vi "Try Step.vi"(8 "error in (no error)":errorcluster, 11 "Future in":refnum<class "Future.lvclass">) -> (0 "error out":errorcluster, 2 "Ready":bool, 3 "Future out":refnum<class "Future.lvclass">)   [LabVIEW 2020, in "Promises.lvlib" / "Future.lvclass"]
doc: "This performs a step of Promise chaining if a value is available and returns as quickly as possible. This VI does no waiting to see if a Promise has been resolved and is meant to return as quickly as possible. Once the last Promise has been resolved, Ready will return as True signifying that a call to <b>Wait.vi</b> will not have to wait for resolution.\n\nNormally promise chaining only happens within a <b>Wait.vi</b> call but this VI allows \"polling\" the value transfer between Promises and return the status of the last Promise in the chain. (Or the status of the only Promise if no <b>Then.vi</b> chaining has been setup."
uses:
  Future.lvclass
  Future.lvclass/Future.ctl
  Promise/Promise.lvclass/Promise.ctl
  Create.vi
  Promise/Promise.lvclass
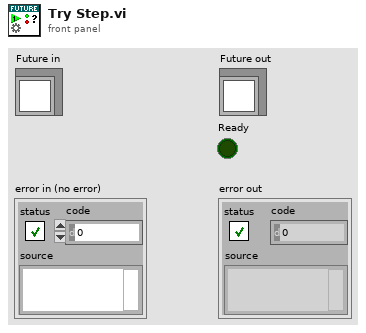
[diagram p1: front panel]
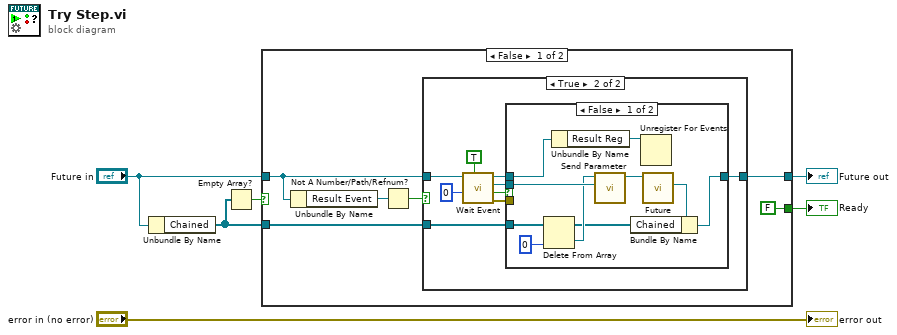
[diagram p0: block diagram]
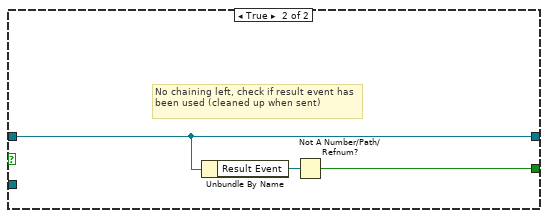
[diagram p4: hidden frame]
diagram:
  n1 = Unbundle By Name("Future in") -> ("Chained"=w2:refnum<class "Promise.lvclass">[])
  n2 = Empty Array?(array=w2) -> (empty?=w3:bool)
  n3 = case shown="False" w3 {
    tunnel: "Future in" -> [w9 w34]
    tunnel: [w12 w34] -> w4
    tunnel: w2 -> [w11 _]
    tunnel: [FALSE w35] -> w1
    frame False {
      n4 = Unbundle By Name(w9) -> ("Result Event"=w8:refnum<user-event>)
      n5 = Not A Number/Path/Refnum?(number/path/refnum=w8) -> (NaN/Path/Refnum?=w7:bool)
      n6 = case shown="True" w7 {
        tunnel: [w13 w17] -> w12
        tunnel: w11 -> [_ w16]
        tunnel: w9 -> [w13 w14]
        frame False {
          # "Han't been fired yet"
        }
        frame True {
          n7 = call "Wait Event.vi"("Keep Event Reg (F)"=TRUE, "Timeout mS (-1)"=0, "Future in"=w14) -> ("error out"=w20:errorcluster, "Timed Out"=w15:bool, "Value"=w18:refnum<class>, "Future out"=w19:refnum<class "Future.lvclass">)  [unwired: 5 in]
          n8 = case shown="False" w15 {
            tunnel: w19 -> [w32 w33]
            tunnel: w18 -> [w30 _]
            tunnel: [w24 w33] -> w17
            tunnel: w16 -> [w28 _]
            tunnel: w20 -> [_ _]
            frame False {
              n9 = Delete From Array(array=w28, index=0) -> (deleted portion=w26:refnum<class "Promise.lvclass">, array with subset deleted=w23:refnum<class "Promise.lvclass">[])  [unwired: 1 in]
              n10 = Unbundle By Name(w32) -> ("Result Reg"=w31:refnum<event-registration>)
              n11 = call "Send Parameter.vi"("Parameter"=w30, "Promise in"=w26) -> ("Promise out"=w29:refnum<class "Promise.lvclass">)  [unwired: 8 in, 1 out]
              n12 = Unregister For Events(event registration refnum=w31) -> ()  [unwired: 1 in, 1 out]
              n13 = call "Future.vi"("Promise in"=w29) -> ("Future"=w25:refnum<class "Future.lvclass">)  [unwired: 9 in, 1 out]
              n14 = Bundle By Name(cluster=w25, "Chained"=w23) -> (w24:refnum<class "Future.lvclass">)
            }
            frame True {
            }
          }
        }
      }
    }
    frame True {
      # "No chaining left, check if result event has been used (cleaned up when sent)"
      n15 = Unbundle By Name(w34) -> ("Result Event"=w36:refnum<user-event>)
      n16 = Not A Number/Path/Refnum?(number/path/refnum=w36) -> (NaN/Path/Refnum?=w35:bool)
    }
  }
  "Future out" <- w4
  "Ready" <- w1
  "error out" <- "error in (no error)"
